vi "S2DS_CreateNewFile.vi"(4 "WC read from file info (in)":T1, 5 "WC from file?":bool, 6 "Script on?":bool, 7 "File info":T2={"File path"=path "", "Header"="", "File name"="", "False channel"=[], "Channel names"=[], "Buffer size"=0, "Format"="%.6f"}) -> (0 "WC read from file info (out)":T1, 1 "Overwrite or create new file?":bool, 2 "Sweep continue?":bool, 3 "File info (out)":T2={"File path"=path "", "Header"="", "File name"="", "False channel"=[], "Channel names"=[], "Buffer size"=0, "Format"="%.6f"})   [LabVIEW 2025]
uses:
  TYPE DEFS/S2DS_Data saving info.ctl
  TYPE DEFS/S2DS_WCFromFileInfo.ctl
  <vilib>/Utility/config.llb/Read Key (U32).vi
  <vilib>/Utility/config.llb/Write Key (U32).vi
  <vilib>/Utility/config.llb/Read Key (String).vi
  <vilib>/Utility/config.llb/Read Key (Path).vi
  <vilib>/Utility/config.llb/Write Key (Path).vi
  <vilib>/Utility/config.llb/NI_LVConfig.lvlib
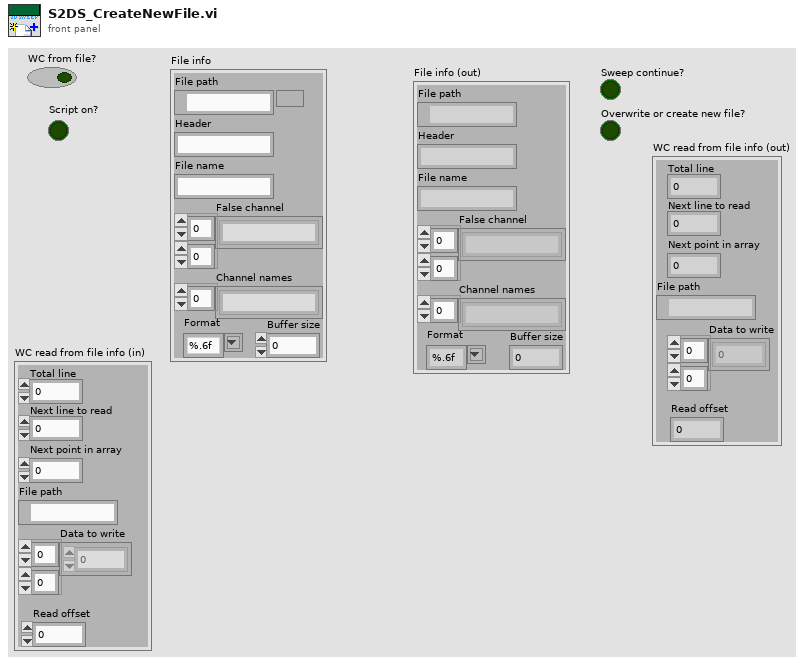
[diagram p1: front panel]
types:
  T1 = typedef "S2DS_WCFromFileInfo.ctl" = cluster{"Next line to read":i32, "Next point in array":i32, "File path":path, "Data to write":dbl[][], "Read offset":i32, "Total line":i32}
  T2 = typedef "S2DS_Data saving info.ctl" = cluster{"File path":path, "Header":string, "File name":string, "False channel":string[][], "Channel names":string[], "Buffer size":i32, "Format":string}
  T3 = typedef "NI_LVConfig.lvlib/Config Data RefNum.ctl" = refnum<k1>
  T4 = enum16{"open", "replace", "create", "open or create", "replace or create", "replace or create with confirmation"}
  T5 = enum16{"Left Button", "Center Button", "Right Button", "Window Close"}
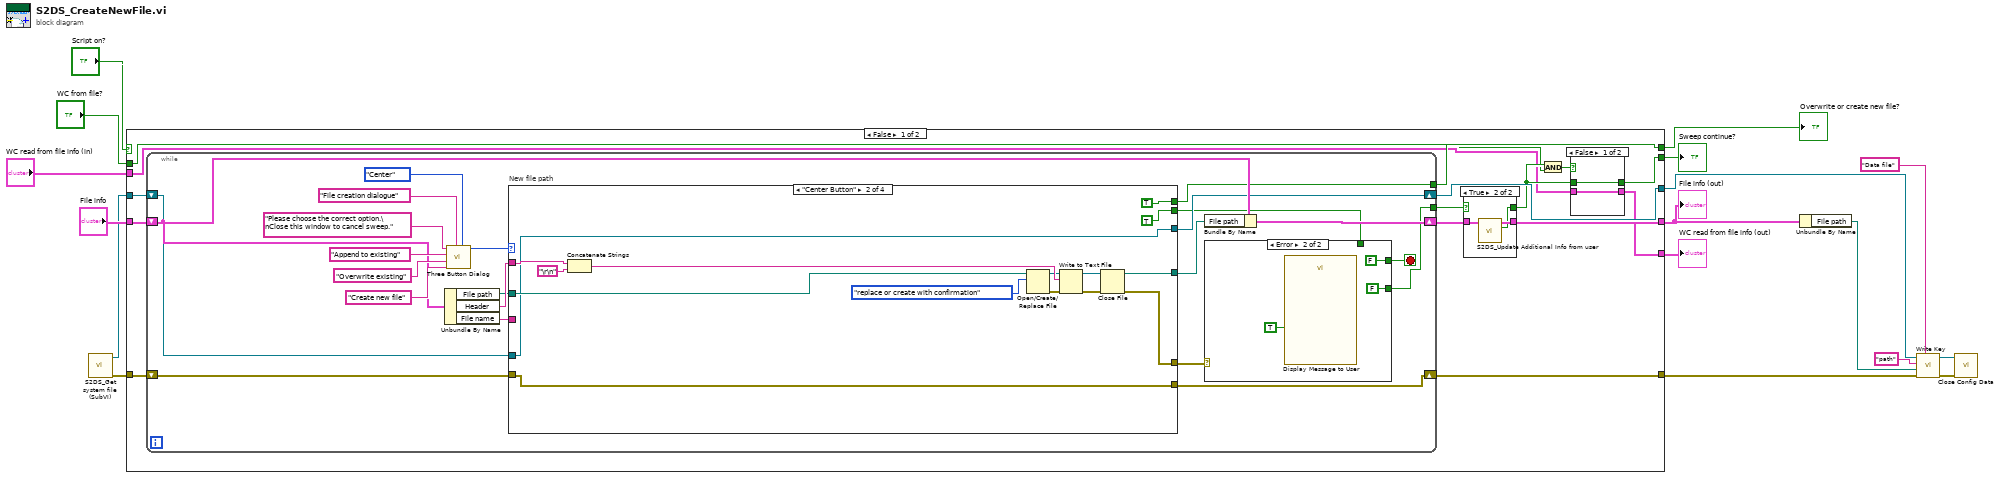
[diagram p0: block diagram]
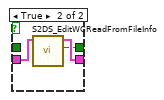
[diagram p2: hidden frame]
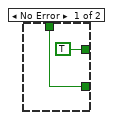
[diagram p4: hidden frame]
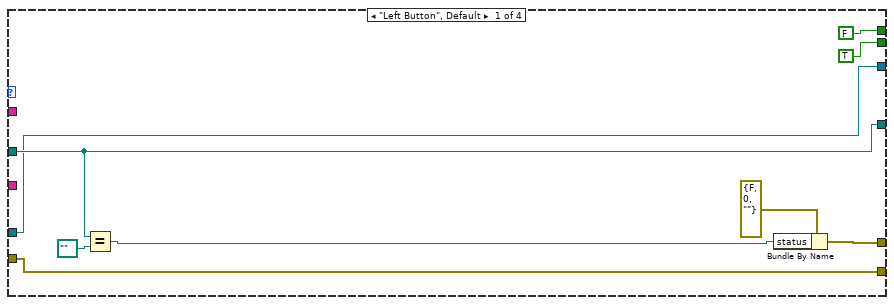
[diagram p5: hidden frame]
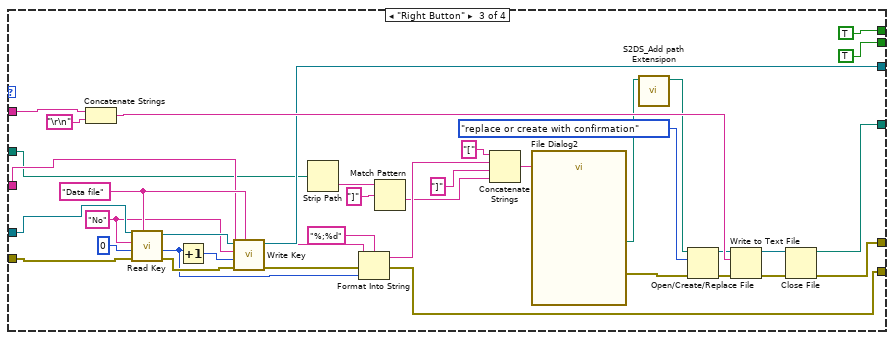
[diagram p6: hidden frame]
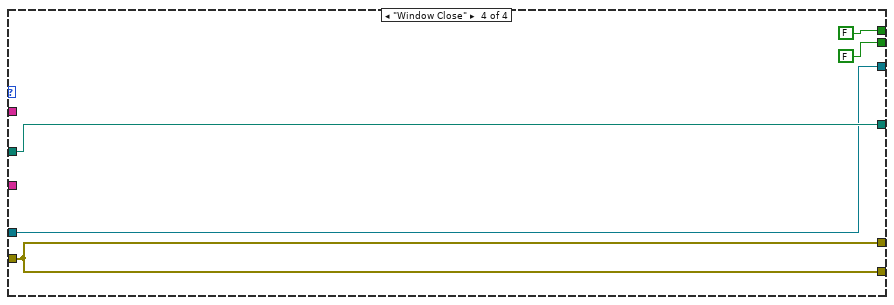
[diagram p7: hidden frame]
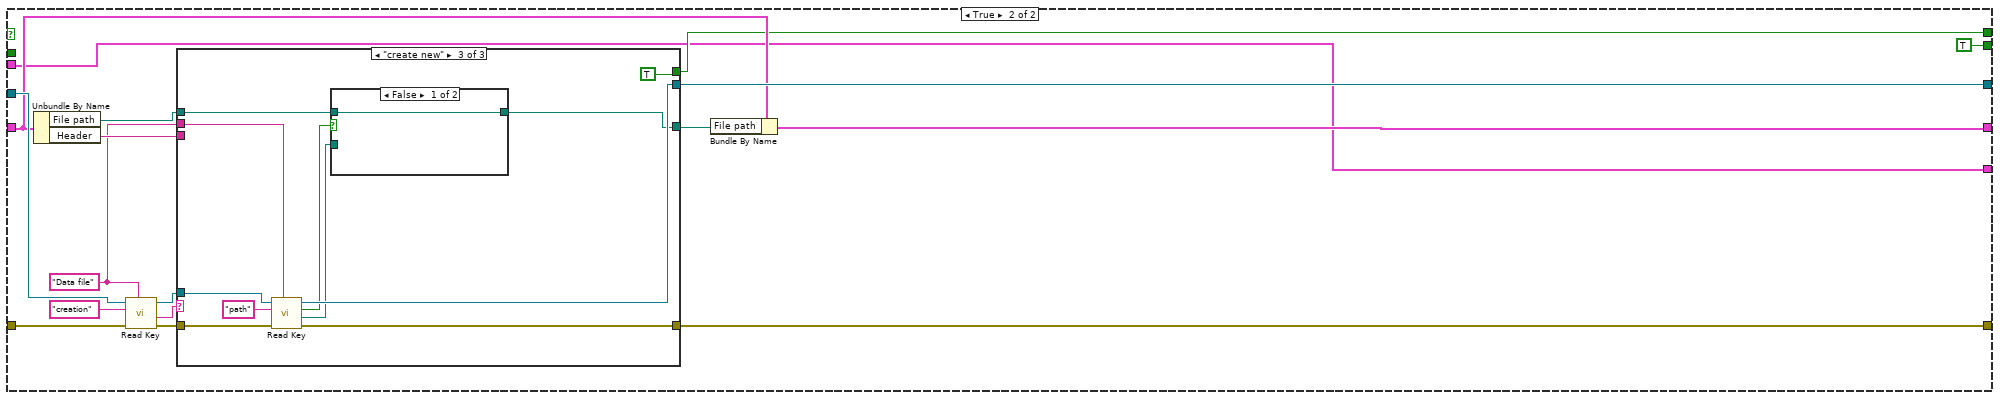
[diagram p8: hidden frame]
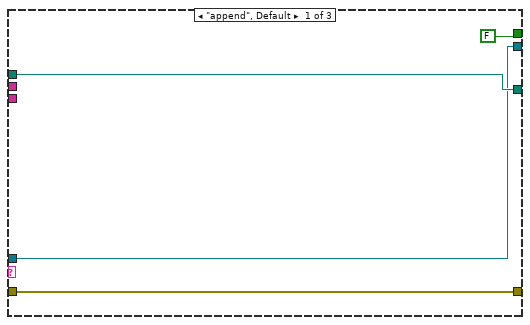
[diagram p9: hidden frame]
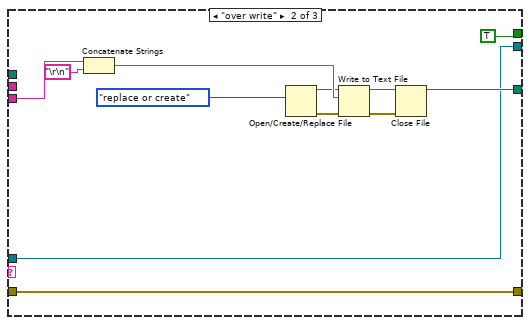
[diagram p10: hidden frame]
diagram:
  n1 = call "S2DS_Get system file (SubVI).vi"() -> ("error out"=w8:errorcluster, "Refnum out"=w9:T3)  [unwired: 10 in]
  n2 = case shown="False" "Script on?" {
    tunnel: "File info" -> [w32 w141]
    tunnel: w9 -> [w29 w145]
    tunnel: w8 -> [w27 w144]
    tunnel: [w26 w143] -> w16
    tunnel: [w28 w142] -> w15
    tunnel: [w30 w139] -> w5
    tunnel: [w25 w138] -> w6
    tunnel: [w22 TRUE] -> w4
    tunnel: [w20 w136] -> w3
    tunnel: "WC read from file info (in)" -> [w19 w136]
    tunnel: "WC from file?" -> [w18 _]
    frame False {
      n3 = while {
        shift-right: [w50] -> w31
        shift-left: w32 -> [w52]
        shift-right: [w48] -> w28
        shift-left: w27 -> [w47]
        shift-right: [w46] -> w26
        shift-left: w29 -> [w49]
        tunnel: [w45] -> w25
        tunnel: [w44] -> w24
        stop <- w53 stop-if-true
        n4 = Unbundle By Name(w52) -> ("File path"=w62:path, "Header"=w63:string, "File name"=w64:string)
        n5 = call <vilib>:"Three Button Dialog.vi"("Justify Message (Left)"=enum16{"Left", "Center", "Right"}."Center", "Window Title (\"\")"="File creation dialogue" ("message"), "Right Button Text (\"Cancel\")"="Create new file" ("Left Button Text (\"Yes\")"), "Center Button Text (\"No\")"="Overwrite existing" ("Center Button Text (\"No\")"), "Left Button Text (\"Yes\")"="Append to existing" ("Right Button Text (\"Cancel\")"), "message"="Please choose the correct option.\nClose this window to cancel sweep.") -> ("Which Button?"=w58:T5)  [unwired: 5 in]
        n6 = case "New file path" shown="\"Center Button\"" w58 {
          tunnel: w64 -> [_ _ w108 _]
          tunnel: w62 -> [w78 w87 w98 w135]
          tunnel: w63 -> [_ w89 w126 _]
          tunnel: [w78 w88 w125 w135] -> w51
          tunnel: [w75 w83 w124 w133] -> w54
          tunnel: w49 -> [w73 w82 w116 w134]
          tunnel: w47 -> [w72 w81 w115 w133]
          tunnel: [w73 w82 w113 w134] -> w46
          tunnel: [w72 w81 w106 w133] -> w48
          tunnel: [FALSE TRUE TRUE FALSE] -> w45
          tunnel: [TRUE TRUE TRUE FALSE] -> w43
          frame "Left Button", Default {
            n7 = Equal?(x=w78, y=path "") -> (x = y?=w74:bool)
            n8 = Bundle By Name(cluster=errorcluster {"status"=FALSE, "code"=0, "source"=""} ("error out"), "status"=w74) -> (w75:errorcluster)
          }
          frame "Center Button" {
            n9 = Concatenate Strings(w89, "\r\n") -> (w90:string)
            n10 = Open/Create/Replace File(file path (use dialog)=w87, operation (0:open)=T4."replace or create with confirmation") -> (refnum out=w84:refnum<file>, error out=w85:errorcluster)  [unwired: 4 in, 1 out]
            n11 = Write to Text File(file (use dialog)=w84, text=w90, error in=w85) -> (refnum out=w93:refnum<file>, error out=w92:errorcluster)  [unwired: 1 in, 1 out]
            n12 = Close File(refnum=w93, error in=w92) -> (path=w88:path, error out=w83:errorcluster)
          }
          frame "Right Button" {
            w110 = "No" ("key")
            w111 = "Data file" ("section")
            n13 = Concatenate Strings(w126, "\r\n") -> (w127:string)
            n14 = call-poly <vilib>:"Read Key.vi"("section"=w111, "error in (no error)"=w115, "default value"=u32 0, "key"=w110, "refnum"=w116) -> ("error out"=w112:errorcluster, "value"=w105:u32, "refnum out"=w114:T3)  [unwired: 3 in, 1 out]
            n15 = Increment(x=w105) -> (x+1=w104:u32)
            n16 = call-poly <vilib>:"Write Key.vi"("section"=w111, "error in (no error)"=w112, "value"=w104, "key"=w110, "refnum"=w114) -> ("error out"=w107:errorcluster, "refnum out"=w113:T3)  [unwired: 4 in, 1 out]
            n17 = Strip Path(path=w98) -> (name=w97:string)  [unwired: 1 out]
            n18 = Format Into String(format string="%;%d", initial string=w108, error in=w107, w105) -> (resulting string=w103:string, error out=w106:errorcluster)
            n19 = Match Pattern(string=w97, regular expression="]") -> (after substring=w95:string)  [unwired: 1 in, 3 out]
            n20 = Concatenate Strings("[" ("string"), w103, "]" ("string"), w95) -> (w100:string)
            n21 = call "File Dialog2"("default name"=w100) -> ("selected path"=w119:path, "error out"=w122:errorcluster)  [unwired: 11 in, 2 out]
            n22 = call "S2DS_Add path Extensipon.vi"("path"=w119) -> ("Path"=w118:path)  [unwired: 10 in]
            n23 = Open/Create/Replace File(file path (use dialog)=w118, error in=w122, operation (0:open)=T4."replace or create with confirmation") -> (refnum out=w123:refnum<file>, error out=w121:errorcluster)  [unwired: 3 in, 1 out]
            n24 = Write to Text File(file (use dialog)=w123, text=w127, error in=w121) -> (refnum out=w130:refnum<file>, error out=w129:errorcluster)  [unwired: 1 in, 1 out]
            n25 = Close File(refnum=w130, error in=w129) -> (path=w125:path, error out=w124:errorcluster)
          }
          frame "Window Close" {
          }
        }
        n26 = Bundle By Name(cluster=w52, "File path"=w51) -> (w50:T2)
        n27 = case shown="Error" w54 {
          tunnel: [TRUE FALSE] -> w53
          tunnel: [w65 FALSE] -> w44
          tunnel: w43 -> [w65 _]
          frame No Error {
          }
          frame Error {
            n28 = call "Display Message to User"("Enable"=TRUE) -> ()  [unwired: 9 in, 2 out]
          }
        }
      }
      n29 = case shown="True" w24 {
        selector: w24 -> [w38 _]
        tunnel: w31 -> [w39 w42]
        tunnel: [w39 w41] -> w30
        tunnel: [w38 w40] -> w21
        frame False {
        }
        frame True {
          n30 = call "S2DS_Update Additional Info from user.vi"("File info (in)"=w42) -> ("OK 2"=w40:bool, "File info (out)"=w41:T2)  [unwired: 9 in]
        }
      }
      n31 = And(x=w21, y=w18) -> (x .and. y?=w23:bool)
      n32 = case shown="False" w23 {
        tunnel: w19 -> [w34 w37]
        tunnel: [w34 w36] -> w20
        tunnel: [w33 w35] -> w22
        tunnel: w21 -> [w33 _]
        frame False {
        }
        frame True {
          n33 = call "S2DS_EditWCReadFromFileInfo.vi"("WC read from file info (out) in"=w37) -> ("Sweep continue"=w35:bool, "WC read from file info (out) out"=w36:T1)  [unwired: 9 in]
        }
      }
    }
    frame True {
      w146 = "Data file" ("section")
      n34 = Unbundle By Name(w141) -> ("File path"=w150:path, "Header"=w149:string)
      n35 = call-poly <vilib>:"Read Key.vi"("section"=w146, "error in (no error)"=w144, "key"="creation", "refnum"=w145) -> ("error out"=w147:errorcluster, "value"=w151:string, "refnum out"=w148:T3)  [unwired: 4 in, 1 out]
      n36 = case shown="\"create new\"" w151 {
        tunnel: w150 -> [w156 _ w172]
        tunnel: [w156 w160 w174] -> w140
        tunnel: w149 -> [_ w161 _]
        tunnel: w148 -> [w155 w159 w179]
        tunnel: [w155 w159 w178] -> w143
        tunnel: w147 -> [w154 w158 w177]
        tunnel: [w154 w158 w176] -> w142
        tunnel: w146 -> [_ _ w171]
        tunnel: [FALSE TRUE TRUE] -> w138
        frame "append", Default {
        }
        frame "over write" {
          n37 = Concatenate Strings(w161, "\r\n") -> (w165:string)
          n38 = Open/Create/Replace File(operation (0:open)=T4."replace or create") -> (refnum out=w162:refnum<file>, error out=w163:errorcluster)  [unwired: 5 in, 1 out]
          n39 = Write to Text File(file (use dialog)=w162, text=w165, error in=w163) -> (refnum out=w168:refnum<file>, error out=w167:errorcluster)  [unwired: 1 in, 1 out]
          n40 = Close File(refnum=w168, error in=w167) -> (path=w160:path)  [unwired: 1 out]
        }
        frame "create new" {
          n41 = call-poly <vilib>:"Read Key.vi"("section"=w171, "error in (no error)"=w177, "key"="path", "refnum"=w179) -> ("error out"=w176:errorcluster, "value"=w173:path, "found?"=w175:bool, "refnum out"=w178:T3)  [unwired: 4 in]
          n42 = case shown="False" w175 {
            tunnel: [w180 w181] -> w174
            tunnel: w173 -> [_ w181]
            tunnel: w172 -> [w180 _]
            frame False {
            }
            frame True {
            }
          }
        }
      }
      n43 = Bundle By Name(cluster=w141, "File path"=w140) -> (w139:T2)
    }
  }
  "File info (out)" <- w5
  "Overwrite or create new file?" <- w6
  "Sweep continue?" <- w4
  "WC read from file info (out)" <- w3
  n44 = Unbundle By Name(w5) -> ("File path"=w7:path)
  n45 = call-poly <vilib>:"Write Key.vi"("section"="Data file", "error in (no error)"=w15, "value"=w7, "key"="path", "refnum"=w16) -> ("error out"=w11:errorcluster, "refnum out"=w12:T3)  [unwired: 4 in, 1 out]
  n46 = call <vilib>:"Close Config Data.vi"("error in (no error)"=w11, "refnum"=w12) -> ()  [unwired: 8 in, 2 out]
